vi "Format Time Stamp.vi"(6 "Time Stamp":timestamp, 8 "error in (no error)":errorcluster, 11 "Application Log in":refnum<class "Application Log.lvclass">) -> (0 "error out":errorcluster, 3 "Application Log out":refnum<class "Application Log.lvclass">, 4 "Formatted Time Stamp":string)   [LabVIEW 2016, in "Stream Log.lvlib" / "Application Log.lvclass"]
doc: "--\nCopyright © 2017 Composed SystemsI All rights reserved.\n\nAuthor: Jon McBee <jon.mcbee@composed.io>\n\nThis library is provided \"AS IS\" ,WITHOUT WARRANTIES OR\nCONDITIONS OF ANY KIND, either express or implied.\n\nComposed Systems -- composed.io\n\nStream 0.0.1.1\nJon McBee - Composed Systems\nCopyright (c) 2017, Composed Systems"
uses:
  <userlib>/Composed Systems/Stream/Log/Application Log/Application Log.lvclass
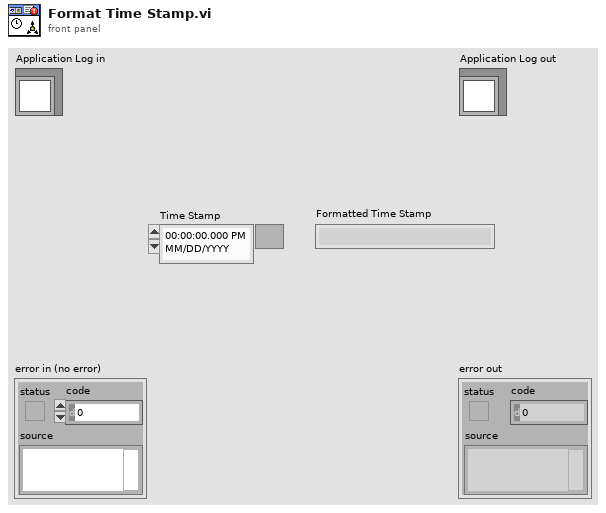
[diagram p1: front panel]
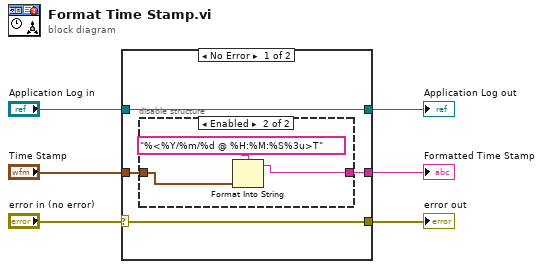
[diagram p0: block diagram]
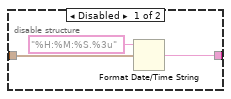
[diagram p2: hidden frame]
diagram:
  n1 = case shown="No Error" "error in (no error)" {
    selector: "error in (no error)" -> [w9 w18]
    tunnel: [w9 w18] -> w5
    tunnel: [w10 w17] -> w3
    tunnel: "Application Log in" -> [w10 w17]
    tunnel: "Time Stamp" -> [w8 _]
    tunnel: [w7 _] -> w1
    frame No Error {
      n2 = disable-structure shown="Enabled" {
        disable-tunnel: w8 -> [w13 w15]
        disable-tunnel: [w11 w14] -> w7
        frame Disabled {
          n3 = Format Date/Time String(time format string (%c)="%H:%M:%S.%3u", seconds (now)=w13) -> (date/time string=w11:string)  [unwired: 1 in]
        }
        frame Enabled {
          n4 = Format Into String(format string="%<%Y/%m/%d @ %H:%M:%S%3u>T", w15) -> (resulting string=w14:string)  [unwired: 2 in, 1 out]
        }
      }
    }
    frame Error {
    }
  }
  "error out" <- w5
  "Application Log out" <- w3
  "Formatted Time Stamp" <- w1
